vi "SW_Load_data_for_Analysis.vi"(0 "Data flow controls":T4, 5 "Cluster of paths input":T3, 9 "Progress bar reference":refnum<vi>, 11 "error in (no error)":errorcluster) -> (1 "Data column names":string[](array[string]), 2 "Absolute timestamp":dbl[](array[numeric]), 3 "Relative timestamp":dbl[](array[numeric]), 4 "X coord":dbl[](array[numeric]), 6 "Y coord":dbl[](array[numeric]), 8 "alpha rot. angle":dbl[](array[numeric]), 10 "Current segment":dbl[](array[numeric]), 12 "Stimulus presets array (loaded)":T1(array[cluster]), 13 "Zones preference array (loaded)":dbl[][](array[numeric]), 14 "Acquisition settings cluster out":T2, 15 "error out":errorcluster)   [LabVIEW 2016]
uses:
  <extravilib>/ChannelInstances/Stream-a[.,.](dbl)/Read With Abort.vi
  <extravilib>/ChannelInstances/Stream-a[.,.](dbl)/Write With Abort.vi
  <extravilib>/ChannelInstances/Stream-a[.,.](dbl)/EndpointRead.vi
  <extravilib>/ChannelInstances/Stream-a[.,.](dbl)/Endpoint.vi
  <vilib>/Utility/file.llb/Read Delimited Spreadsheet (string).vi
  <extravilib>/ChannelInstances/Stream-a[.,.](dbl)/Instantiate.vi
  <extravilib>/ChannelInstances/Stream-a[.,.](dbl)/)Channel.vi
  <resource>/ChannelSupport/_ChannelSupport/WaitIfNeeded.vi
  <vilib>/Utility/config.llb/NI_LVConfig.lvlib
  <extravilib>/ChannelInstances/Stream-a[.,.](dbl).lvlib
panel:
  out "Settings loaded OK":bool
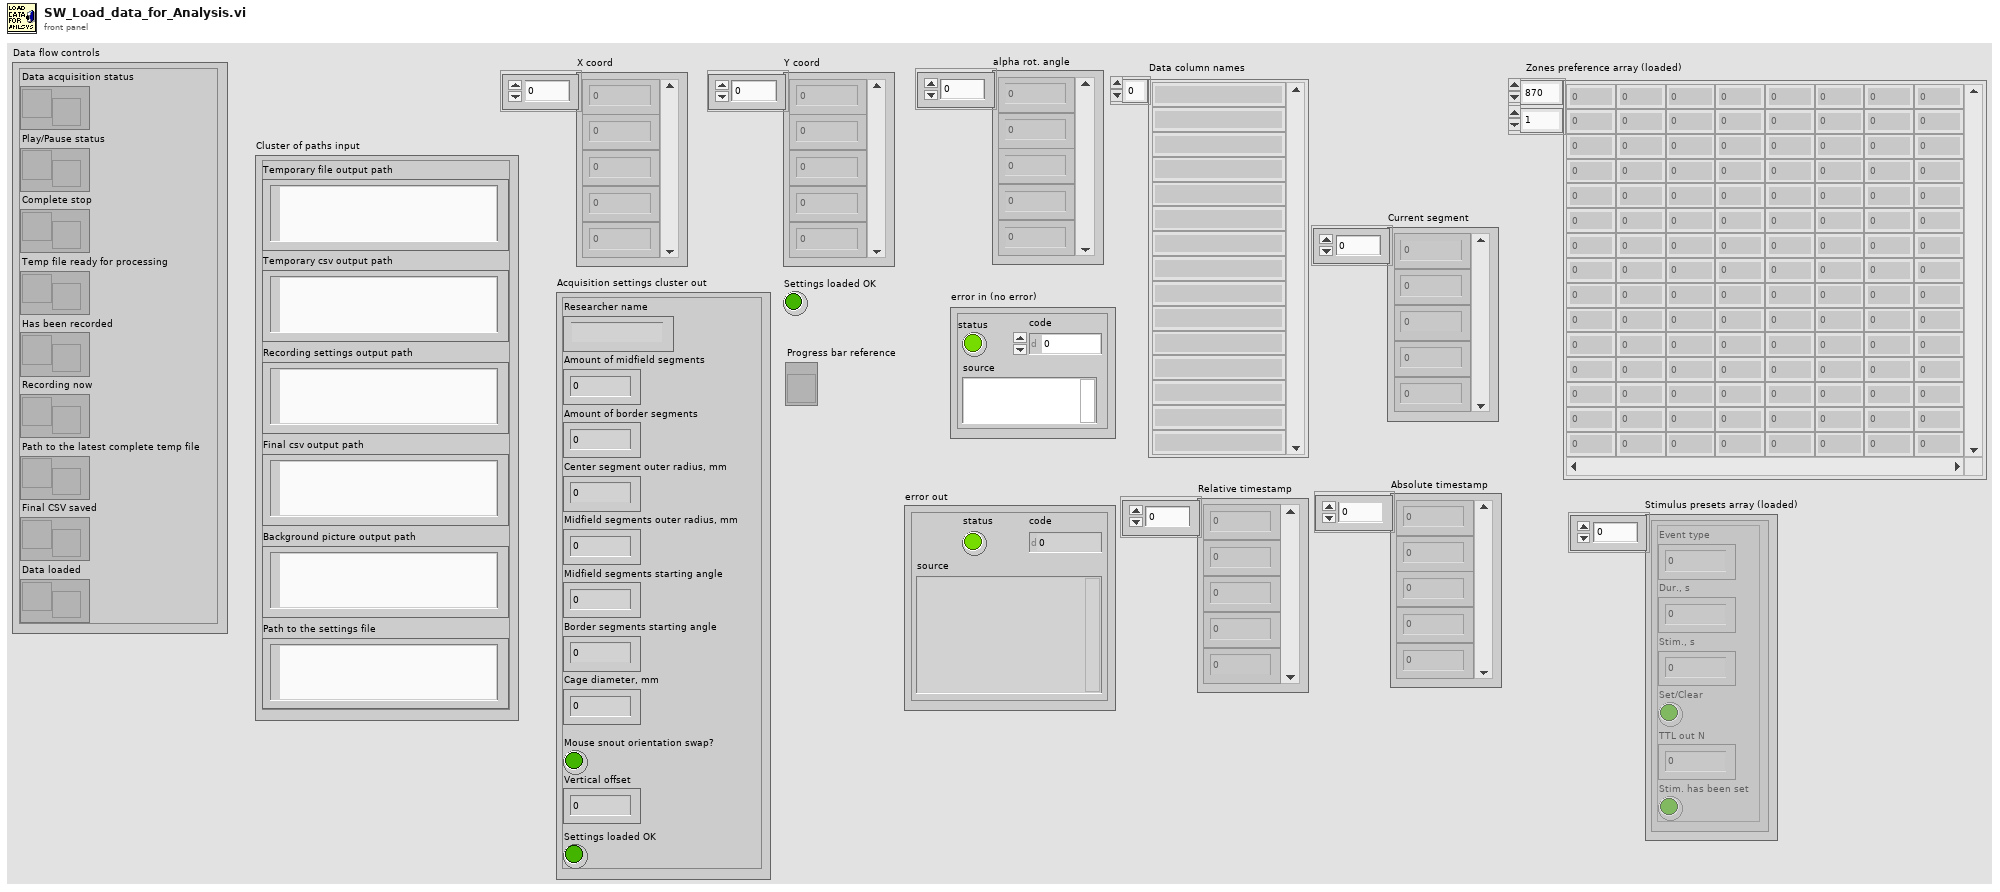
[diagram p1: front panel]
types:
  T1 = cluster{"Event type":u16, "Dur., s":sgl, "Stim., s":sgl, "Set/Clear":bool, "TTL out N":u16, "Stim. has been set":bool}[]
  T2 = cluster{"Researcher name":string, "Amount of midfield segments":u32, "Amount of border segments":u32, "Center segment outer radius, mm":u32, "Midfield segments outer radius, mm":u32, "Midfield segments starting angle":i32, "Border segments starting angle":i32, "Cage diameter, mm":u32, "Mouse snout orientation swap?":bool, "Vertical offset":dbl, "Settings loaded OK":bool}
  T3 = cluster{"Temporary file output path":path, "Temporary csv output path":path, "Recording settings output path":path, "Final csv output path":path, "Background picture output path":path, "Path to the settings file":path}
  T4 = cluster{"Data acquisition status":refnum<notifier>, "Play/Pause status":refnum<notifier>, "Complete stop":refnum<notifier>, "Temp file ready for processing":refnum<notifier>, "Has been recorded":refnum<notifier>, "Recording now":refnum<notifier>, "Path to the latest complete temp file":refnum<notifier>, "Final CSV saved":refnum<notifier>, "Data loaded":refnum<notifier>}
  T5 = typedef "NI_LVConfig.lvlib/Config Data RefNum.ctl" = refnum<k1>
  T6 = typedef "Stream-a[.,.](dbl).lvlib/)Channel.ctl" = refnum<queue>
  T7 = cluster{"Event type":u16, "Cond., s":sgl, "Stim., s":sgl, "Set/Clear":bool, "TTL out N":u16, "Stim. has been set":bool}
  T8 = cluster{"Event type":u16, "Dur., s":sgl, "Stim., s":sgl, "Set/Clear":bool, "TTL out N":u16, "Stim. has been set":bool}
  T9 = cluster{"value":string, "value":u32, "value":u32, "value":u32, "value":u32, "value":i32, "value":i32, "value":u32, "value":bool, "value":dbl, bool}
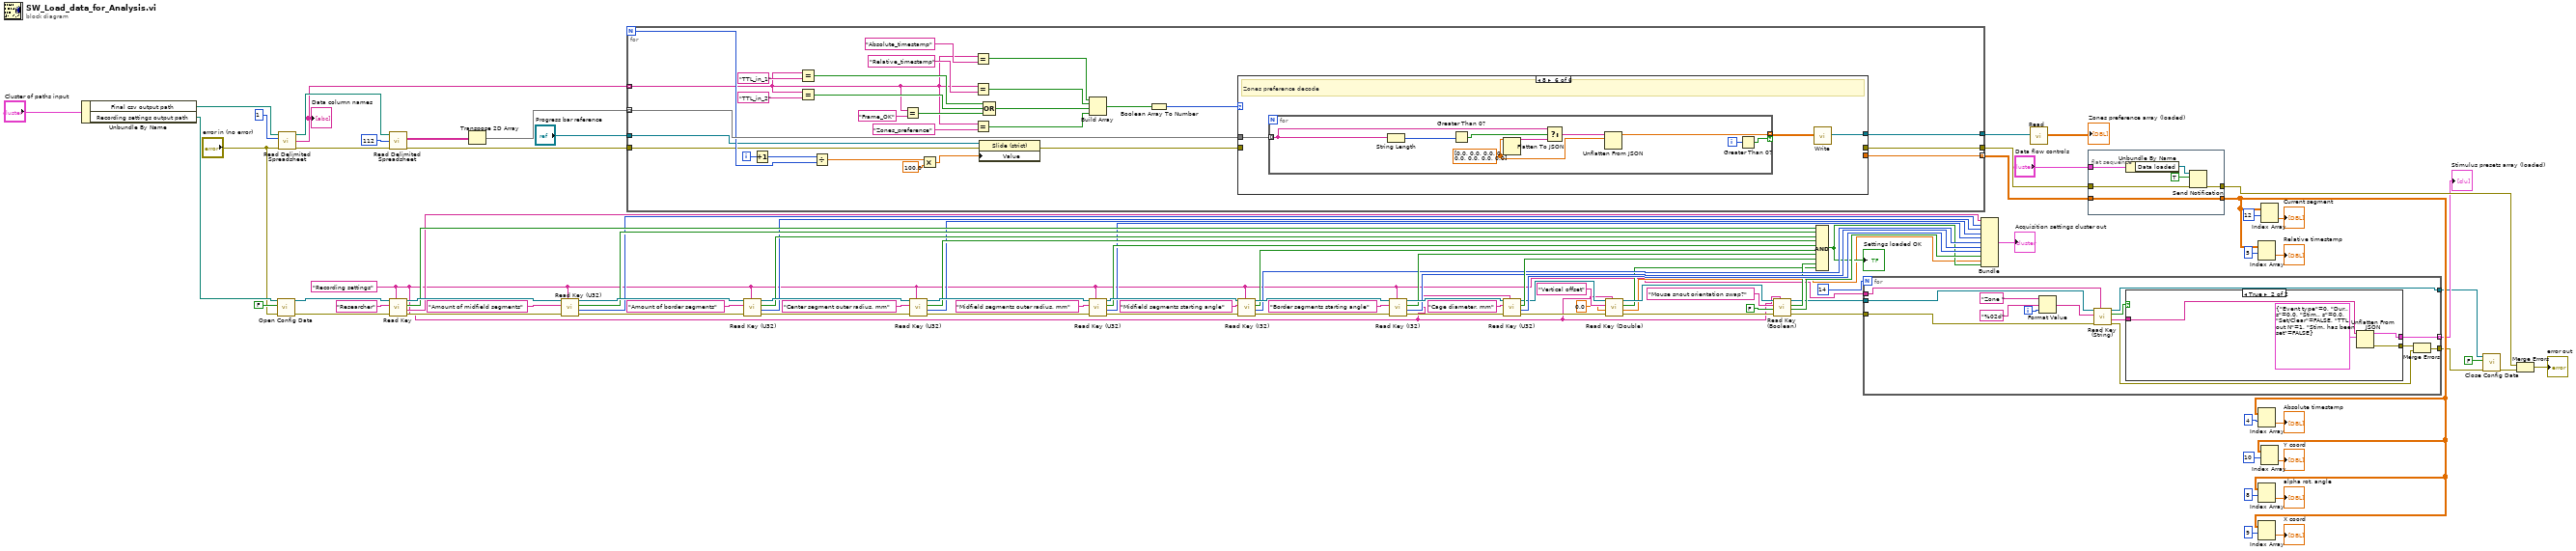
[diagram p0: block diagram]
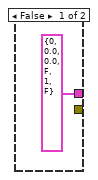
[diagram p2: hidden frame]
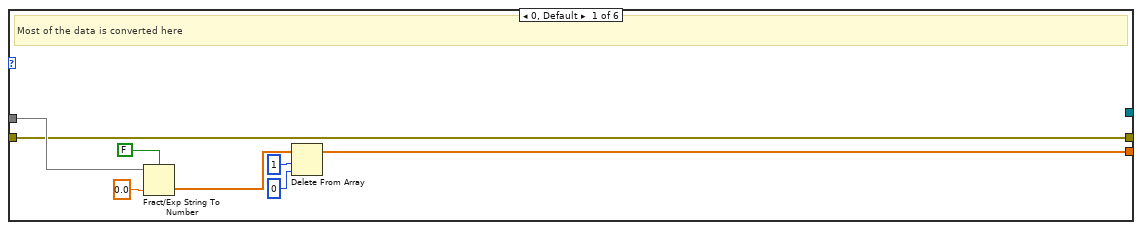
[diagram p3: hidden frame]
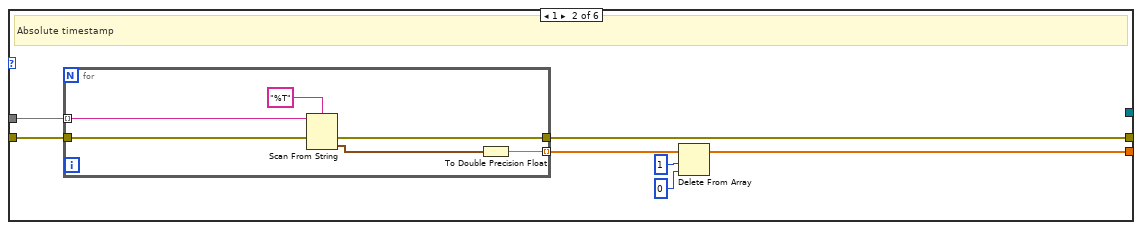
[diagram p4: hidden frame]
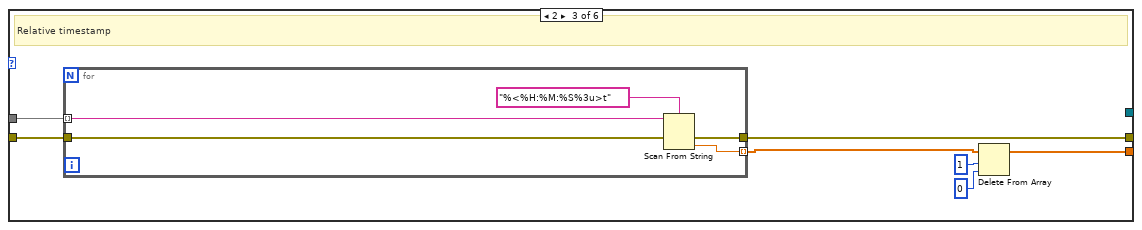
[diagram p5: hidden frame]
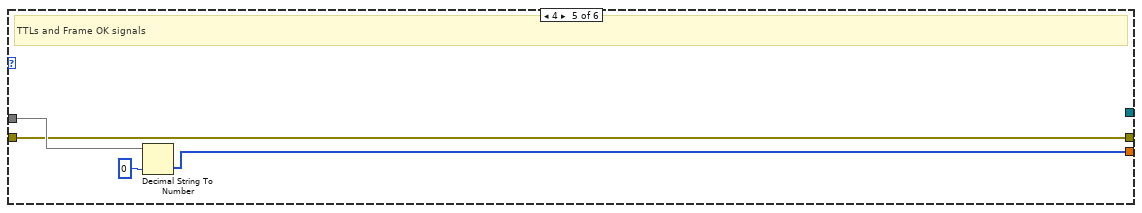
[diagram p7: hidden frame]
diagram:
  w3 = "Recording settings" ("section")
  n1 = Unbundle By Name("Cluster of paths input") -> ("Final csv output path"=w90:path, "Recording settings output path"=w78:path)
  n2 = call <vilib>:"Open Config Data.vi"("error in (no error)"="error in (no error)", "create file if necessary (T)"=FALSE, "configuration file path"=w78) -> ("error out"=w53:errorcluster, "refnum"=w76:T5)  [unwired: 6 in, 1 out]
  n3 = call-poly <vilib>:"Read Delimited Spreadsheet.vi"("file path (dialog if empty)"=w90, "number of rows (all:-1)"=1, "error in (no error)"="error in (no error)") -> ("new file path (Not A Path if cancelled)"=w92:path, "first row"=w19:string[], "error out"=w95:errorcluster)  [unwired: 7 in, 3 out]
  "Data column names" <- w19
  n4 = call-poly <vilib>:"Read Delimited Spreadsheet.vi"("file path (dialog if empty)"=w92, "start of read offset (chars.:0)"=112, "error in (no error)"=w95) -> ("all rows"=w93:string[][], "error out"=w83:errorcluster)  [unwired: 7 in, 4 out]
  n5 = call-poly <vilib>:"Read Key.vi"("section"=w3, "error in (no error)"=w53, "key"="Researcher", "refnum"=w76) -> ("error out"=w72:errorcluster, "value"=w39:string, "found?"=w52:bool, "refnum out"=w74:T5)  [unwired: 4 in]
  n6 = Transpose 2D Array(2D array=w93) -> (transposed array=w91:string[][])
  n7 = call <vilib>:"Read Key (U32).vi"("section"=w3, "error in (no error)"=w72, "key"="Amount of midfield segments", "refnum"=w74) -> ("error out"=w70:errorcluster, "value"=w38:u32, "found?"=w51:bool, "refnum out"=w71:T5)  [unwired: 4 in]
  n8 = for {
    N -> [w110]
    tunnel: w19 -> [w100] mode=indexing
    tunnel: w91 -> [w115] mode=indexing
    tunnel: [w112] -> w81 mode=indexing
    tunnel: w83 -> [w103]
    tunnel: [w106] -> w82
    tunnel: "Progress bar reference" -> [w104]
    tunnel: [w98] -> w18
    i -> [w111]
    n9 = Increment(x=w111) -> (x+1=w107:i32)
    n10 = Equal?(x=w100, y="TTL_in_1") -> (x = y?=w121:bool)
    n11 = Equal?(x=w100, y="TTL_in_2") -> (x = y?=w120:bool)
    n12 = Divide(x=w107, y=w110) -> (x/y=w109:dbl)
    n13 = Equal?(x=w100, y="Frame_OK") -> (x = y?=w119:bool)
    n14 = Multiply(x=w109, y=100.0) -> (x*y=w105:dbl)
    n15 = Equal?(x=w100, y="Absolute_timestamp") -> (x = y?=w113:bool)
    n16 = Equal?(x=w100, y="Relative_timestamp") -> (x = y?=w114:bool)
    n17 = Equal?(x=w100, y="Zones_preference") -> (x = y?=w99:bool)
    n18 = property on="Property Node" class="Slide (strict)"(reference=w104, error in=w103, "Value"=w105) -> (error out=w102:errorcluster)  [unwired: 1 out]
    n19 = Compound Arithmetic op=OR(w121, w120, w119) -> (w118:bool)
    n20 = Build Array(w113, w114, w118, w99) -> (w117:bool[])
    n21 = Boolean Array To Number(Boolean array=w117) -> (number=w116:u32)
    n22 = case shown="8" w116 {
      tunnel: w115 -> [w134 w141 w154 _ w164 w167]
      tunnel: [w127 w135 w148 _ w162 _] -> w112
      tunnel: w102 -> [w131 w140 w153 w160 w161 _]
      tunnel: [w131 w139 w152 w160 w161 _] -> w106
      tunnel: [_ _ _ _ _ w165] -> w98
      frame 0, Default {
        # "Most of the data is converted here"
        n23 = Fract/Exp String To Number(use system decimal point (T)=FALSE, string=w134, default (0 dbl)=0.0 ("default (0 DBL)")) -> (number=w130:dbl[])  [unwired: 1 in, 1 out]
        n24 = Delete From Array(array=w130, length=1, index=0) -> (array with subset deleted=w127:dbl[])  [unwired: 1 out]
      }
      frame 1 {
        # "Absolute timestamp"
        n25 = for {
          tunnel: w141 -> [w146] mode=indexing
          tunnel: [w144] -> w136 mode=indexing
          tunnel: w140 -> [w143]
          tunnel: [w142] -> w139
          n26 = Scan From String(format string="%T", input string=w146, error in=w143) -> (error out=w142:errorcluster, output 1=w145:timestamp)  [unwired: 2 in, 2 out]
          n27 = To Double Precision Float(number=w145) -> (double precision float=w144:dbl)
        }
        n28 = Delete From Array(array=w136, length=1, index=0) -> (array with subset deleted=w135:dbl[])  [unwired: 1 out]
      }
      frame 2 {
        # "Relative timestamp"
        n29 = for {
          tunnel: w154 -> [w158] mode=indexing
          tunnel: [w157] -> w149 mode=indexing
          tunnel: w153 -> [w156]
          tunnel: [w155] -> w152
          n30 = Scan From String(format string="%<%H:%M:%S%3u>t", input string=w158, error in=w156) -> (error out=w155:errorcluster, output 1=w157:dbl)  [unwired: 2 in, 2 out]
        }
        n31 = Delete From Array(array=w149, length=1, index=0) -> (array with subset deleted=w148:dbl[])  [unwired: 1 out]
      }
      frame 3 {
      }
      frame 4 {
        # "TTLs and Frame OK signals"
        n32 = Decimal String To Number(string=w164, default (0L)=u8 0 ("default (0 I32)")) -> (number=w162:u8[])  [unwired: 1 in, 1 out]
      }
      frame 8 {
        # "Zones preference decode"
        n33 = for {
          tunnel: w167 -> [w173] mode=indexing
          tunnel: [w170] -> w166 mode=indexing if=w169
          i -> [w168]
          w171 = dbl[] [0.0, 0.0, 0.0, 0.0, 0.0, 0.0, 0.0, 0.0, 0.0] ("Zones normalized allocation array")
          n34 = String Length(string=w173) -> (length=w176:i32)
          n35 = Greater Than 0?(x=w176) -> (x > 0?=w175:bool)
          n36 = Flatten To JSON(anything=w171) -> (JSON string=w172:string)  [unwired: 2 in, 1 out]
          n37 = Select(t=w173, s=w175, f=w172) -> (s? t:f=w174:string)
          n38 = Unflatten From JSON(JSON string=w174, type and defaults=w171) -> (value=w170:dbl[])  [unwired: 5 in, 1 out]
          n39 = Greater Than 0?(x=w168) -> (x > 0?=w169:bool)
        }
        n40 = call <extravilib>:"Write.vi"("element"=w166) -> ("channel"=w165:T6)  [unwired: 8 in, 2 out]
      }
    }
  }
  n41 = call <vilib>:"Read Key (U32).vi"("section"=w3, "error in (no error)"=w70, "key"="Amount of border segments", "refnum"=w71) -> ("error out"=w68:errorcluster, "value"=w37:u32, "found?"=w50:bool, "refnum out"=w61:T5)  [unwired: 4 in]
  n42 = call <vilib>:"Read Key (U32).vi"("section"=w3, "error in (no error)"=w68, "key"="Center segment outer radius, mm", "refnum"=w61) -> ("error out"=w67:errorcluster, "value"=w36:u32, "found?"=w49:bool, "refnum out"=w60:T5)  [unwired: 4 in]
  n43 = call <vilib>:"Read Key (U32).vi"("section"=w3, "error in (no error)"=w67, "key"="Midfield segments outer radius, mm", "refnum"=w60) -> ("error out"=w66:errorcluster, "value"=w35:u32, "found?"=w48:bool, "refnum out"=w59:T5)  [unwired: 4 in]
  n44 = call <vilib>:"Read Key (I32).vi"("section"=w3, "error in (no error)"=w66, "key"="Midfield segments starting angle", "refnum"=w59) -> ("error out"=w65:errorcluster, "value"=w34:i32, "found?"=w47:bool, "refnum out"=w58:T5)  [unwired: 4 in]
  n45 = call <vilib>:"Read Key (I32).vi"("section"=w3, "error in (no error)"=w65, "key"="Border segments starting angle", "refnum"=w58) -> ("error out"=w64:errorcluster, "value"=w33:i32, "found?"=w46:bool, "refnum out"=w57:T5)  [unwired: 4 in]
  n46 = call <vilib>:"Read Key (U32).vi"("section"=w3, "error in (no error)"=w64, "key"="Cage diameter, mm", "refnum"=w57) -> ("error out"=w16:errorcluster, "value"=w32:u32, "found?"=w45:bool, "refnum out"=w14:T5)  [unwired: 4 in]
  n47 = call <vilib>:"Read Key (Double).vi"("section"=w3, "error in (no error)"=w16, "default value"=0.0, "key"="Vertical offset", "refnum"=w14) -> ("error out"=w15:errorcluster, "value"=w8:dbl, "found?"=w10:bool, "refnum out"=w13:T5)  [unwired: 3 in]
  n48 = call <vilib>:"Read Key (Boolean).vi"("section"=w3, "error in (no error)"=w15, "default value"=FALSE, "key"="Mouse snout orientation swap?", "refnum"=w13) -> ("error out"=w5:errorcluster, "value"=w25:bool, "found?"=w26:bool, "refnum out"=w2:T5)  [unwired: 3 in]
  n49 = Compound Arithmetic op=AND(w52, w51, w50, w49, w48, w47, w46, w45, w26, w10) -> (w9:bool)
  "Settings loaded OK" <- w9
  n50 = for {
    N: 14 -> [_]
    tunnel: w2 -> [w188]
    tunnel: [w187] -> w1
    tunnel: w3 -> [w186]
    tunnel: w5 -> [w184]
    tunnel: [w178] -> w4
    tunnel: [w181] -> w6 mode=indexing
    i -> [w179]
    n51 = Format Value(string ("")="Zone ", format string="%02d", value (0)=w179) -> (output string=w185:string)
    n52 = call <vilib>:"Read Key (String).vi"("section"=w186, "error in (no error)"=w184, "key"=w185, "refnum"=w188) -> ("error out"=w183:errorcluster, "value"=w182:string, "found?"=w180:bool, "refnum out"=w187:T5)  [unwired: 4 in]
    n53 = case shown="True" w180 {
      tunnel: w182 -> [_ w195]
      tunnel: [T7 {"Event type"=0, "Cond., s"=0.0, "Stim., s"=0.0, "Set/Clear"=FALSE, "TTL out N"=1, "Stim. has been set"=FALSE} ("Cluster of the stimuls settings") w194] -> w181
      tunnel: [_ w193] -> w177
      frame False {
      }
      frame True {
        n54 = Unflatten From JSON(JSON string=w195, type and defaults=T8 {"Event type"=0, "Dur., s"=0.0, "Stim., s"=0.0, "Set/Clear"=FALSE, "TTL out N"=1, "Stim. has been set"=FALSE} ("Cluster of the stimuls settings")) -> (value=w194:T8, error out=w193:errorcluster)  [unwired: 5 in]
      }
    }
    n55 = Merge Errors(w177, w183) -> (w178:errorcluster)
  }
  "Stimulus presets array (loaded)" <- w6
  n56 = Bundle("value"=w39, "value"=w38, "value"=w37, "value"=w36, "value"=w35, "value"=w34, "value"=w33, "value"=w32, "value"=w25, "value"=w8, w9) -> (→"Acquisition settings cluster out":T9)  [unwired: 1 in]
  n57 = call <extravilib>:"Read.vi"("channel"=w18) -> ("element"=→"Zones preference array (loaded)":dbl[][])  [unwired: 6 in, 4 out]
  n58 = flat-sequence {
    tunnel: w81 -> [w201]
    tunnel: [w201] -> w20
    tunnel: "Data flow controls" -> [w198]
    tunnel: [w197] -> w63
    tunnel: w82 -> [w196]
    frame #0 {
      n59 = Unbundle By Name(w198) -> ("Data loaded"=w199:refnum<notifier>)
      n60 = Send Notification(notification=TRUE, notifier=w199, error in (no error)=w196) -> (error out=w197:errorcluster)  [unwired: 1 out]
    }
  }
  n61 = Index Array(array=w20, index (row)=5 ("disabled index (col)")) -> (element=→"Relative timestamp":dbl[])  [unwired: 1 in]
  n62 = Index Array(array=w20, index (row)=4 ("disabled index (col)")) -> (element=→"Absolute timestamp":dbl[])  [unwired: 1 in]
  n63 = Index Array(array=w20, index (row)=8) -> (element=→"alpha rot. angle":dbl[])  [unwired: 1 in]
  n64 = Index Array(array=w20, index (row)=9 ("disabled index (col)")) -> (element=→"X coord":dbl[])  [unwired: 1 in]
  n65 = Index Array(array=w20, index (row)=12) -> (element=→"Current segment":dbl[])  [unwired: 1 in]
  n66 = Index Array(array=w20, index (row)=10) -> (element=→"Y coord":dbl[])  [unwired: 1 in]
  n67 = call <vilib>:"Close Config Data.vi"("error in (no error)"=w4, "write file if changed (T)"=FALSE, "refnum"=w1) -> ("error out"=w56:errorcluster)  [unwired: 7 in, 1 out]
  n68 = Merge Errors(w63, w56) -> (→"error out":errorcluster)
